vi "ABB Test Locked Rotor.vi"() -> ()   [LabVIEW 2017]
uses:
  Temp error msg.ctl
  Video Display Buttons.ctl
  ABB global.vi
panel:
  in  "Video Displays":T1
  in  "Temp error":T2="Error: Temperature measurement "
  out "Auto Readings":cluster{"%":dbl[], "Recorded":bool[]}
  in  "Simulate I":dbl(slide)
  out "Readings":string[][](table)
  out "In Range?":bool[](array[boolean])
  out "saved Readings":dbl[][](array[numeric])
  out "% rated current":dbl format="%.1f"
  out "Rated Current":dbl
  out "Serial number":string
  out "W.O number":string
  out "Power":string[][](table)
  out "Current & Voltage":string[][](table)
  out "Norma 5000 Error":string
  in  "Record":bool
  out "Readings":string[][](table)
  in  "View":enum16{"Graph", "Readings"}(ring)
  out "Number readings":i32
  out "Status":enum16{"Stopped", "Running"}(ring)
  out "Timedate":string
  in  "End test":bool
  in  "Start":bool
  in  "Read Mode":enum16{"Auto", "Manual"}(ring)
  in  "Exit":bool
  out "Current vs Voltage":T3(graph)
  # "Locked Rotor Test"
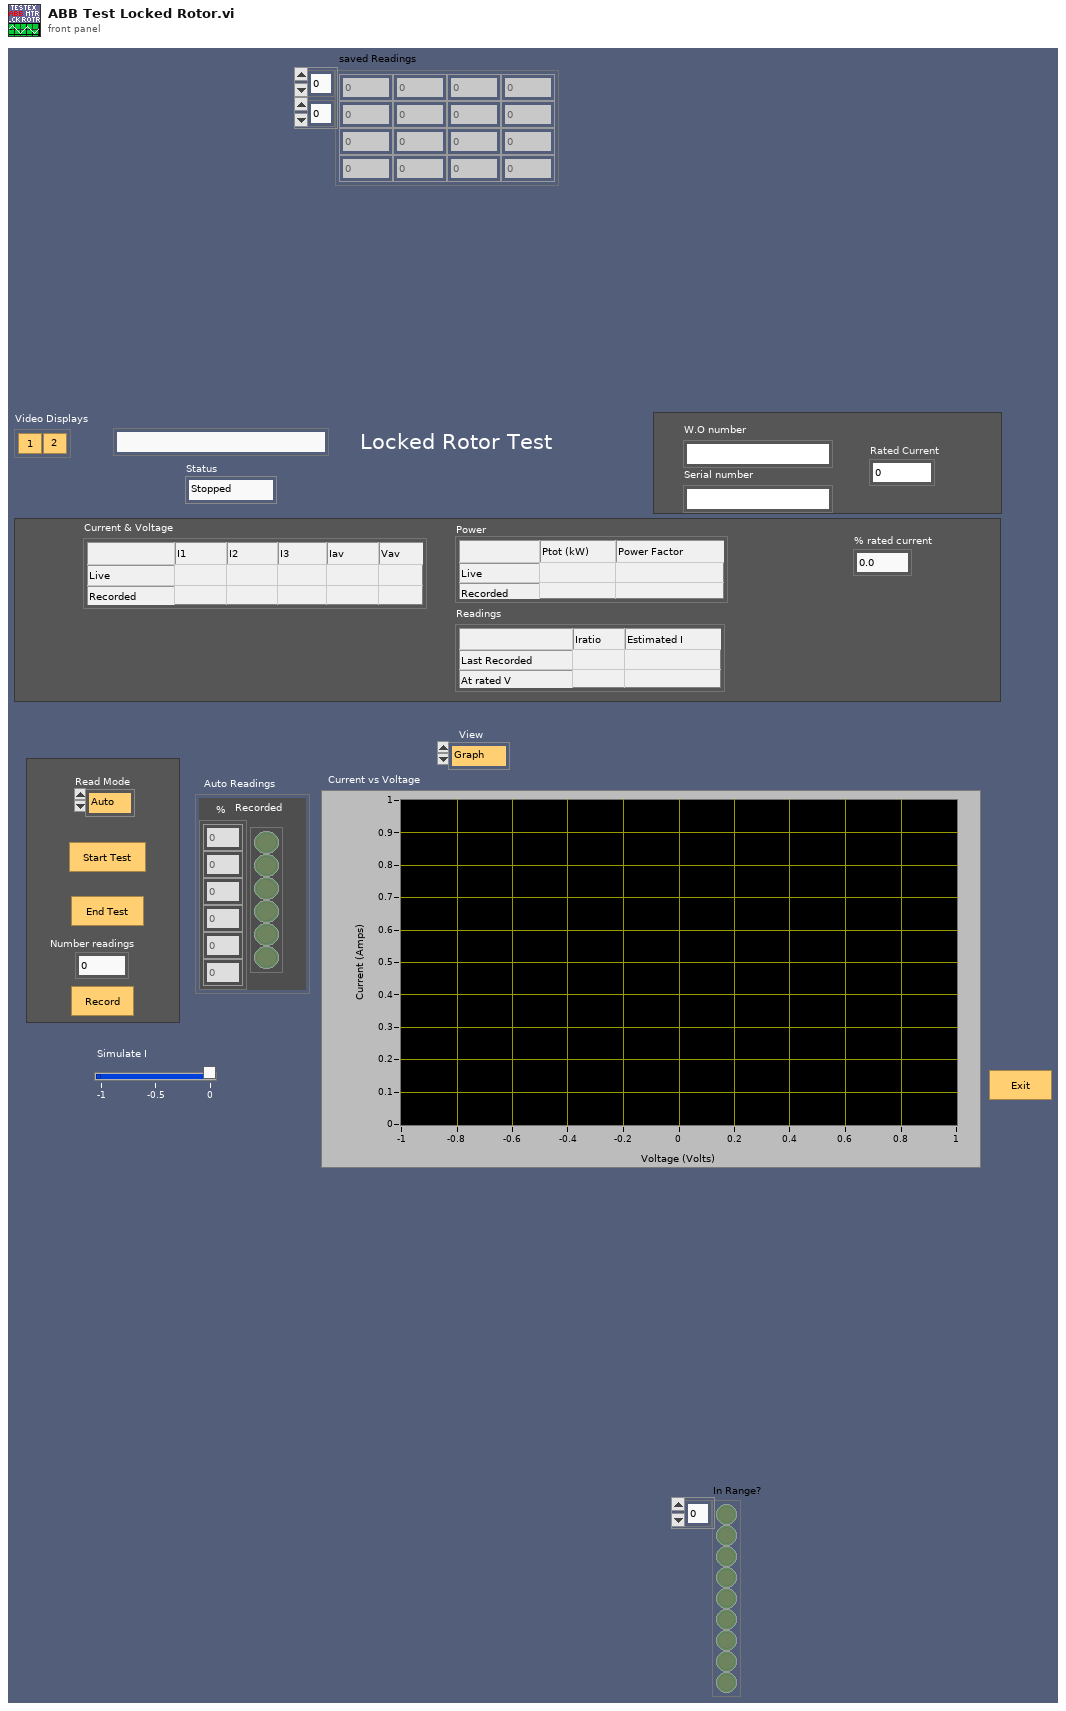
[diagram p1: front panel]
types:
  T1 = typedef "Video Display Buttons.ctl" = cluster{"1":bool, "1 2":bool}
  T2 = typedef "Temp error msg.ctl" = string
  T3 = cluster{"Sorted 2D Array":dbl[], "Sorted 2D Array":dbl[]}
  T4 = cluster{"Voltage":dbl, "Power":dbl, "Current":dbl, "PF":dbl}
  T5 = cluster{"VT Primary":dbl, "VT Secondary":dbl, "CT  Primary":dbl, "CT Secondary":dbl, "Current Shunt":enum16{"Internal", "External"}, "Avg interval":dbl}
  T6 = cluster{"VT Primary":dbl, "VT Secondary":dbl, "CT  Primary":dbl, "CT Secondary":dbl, "Current Shunt":enum16{"Internal", "External"}, "Averaging interval (secs)":dbl}
  T7 = cluster{"Visa sesssion":refnum<visa-resource-name>, "error":errorcluster}
  T8 = cluster{"Simulate Norma":bool, "Norma 5000 Address":u8, "WebDaq IP Address":string, "Simulate cDAQ":bool}
  T9 = cluster{"Number Values":i32, "Tolerance":dbl, "Value (ratio) ":dbl[], "Hold time (sec)":dbl}
  T10 = cluster{"V":dbl, "A":dbl, "W":dbl, "VA":dbl, "VAr":dbl, "Pf":dbl}
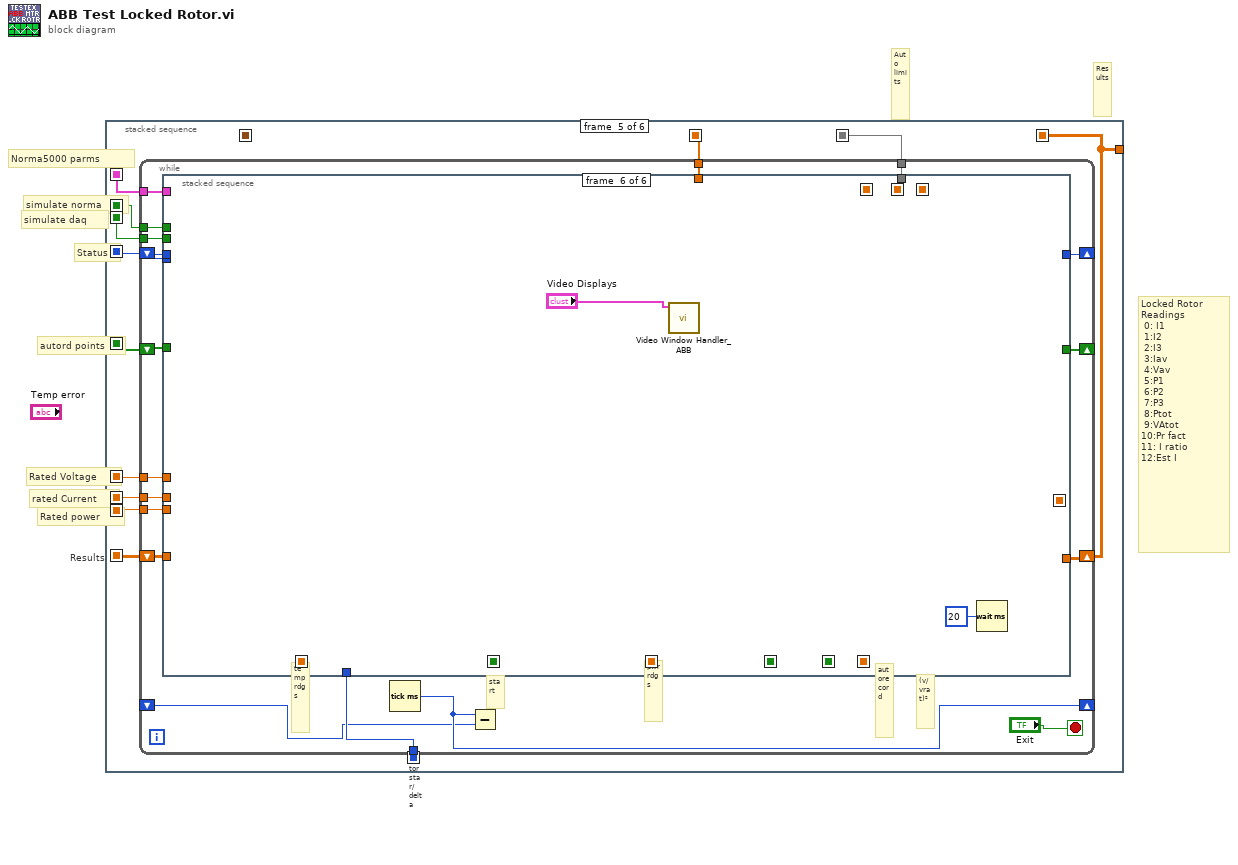
[diagram p0: block diagram]
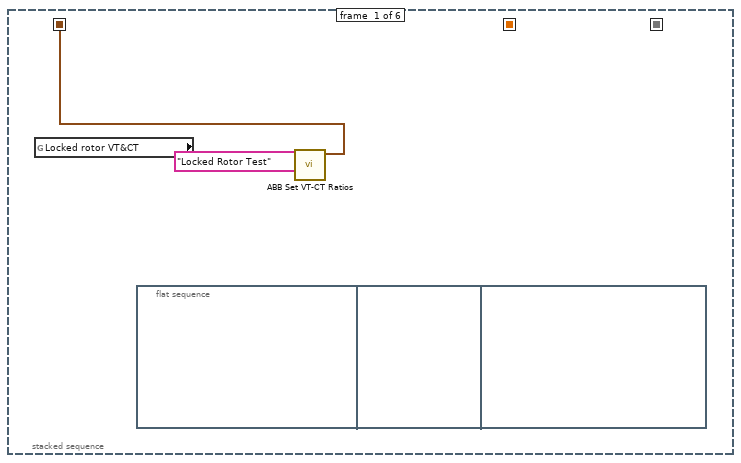
[diagram p2: hidden frame]
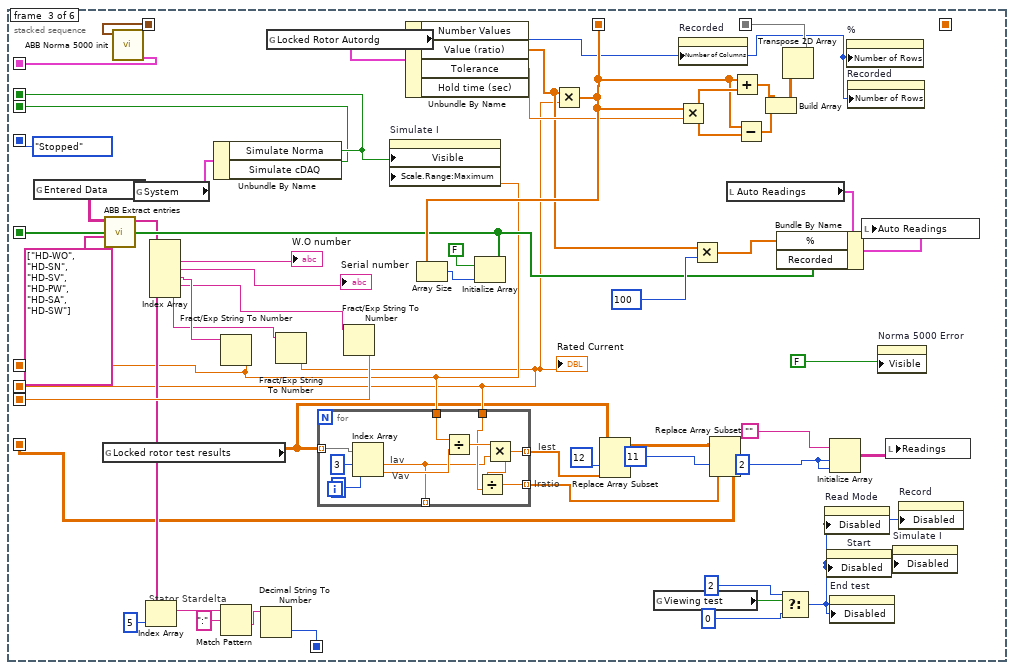
[diagram p4: hidden frame]
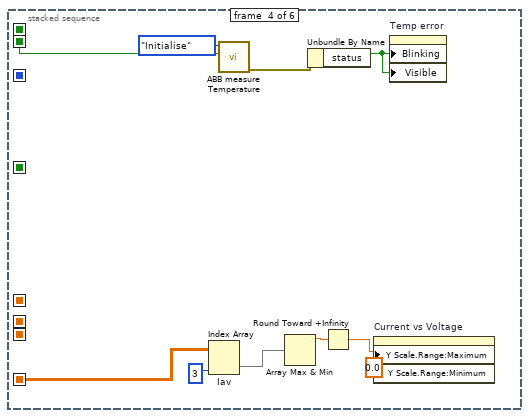
[diagram p5: hidden frame]
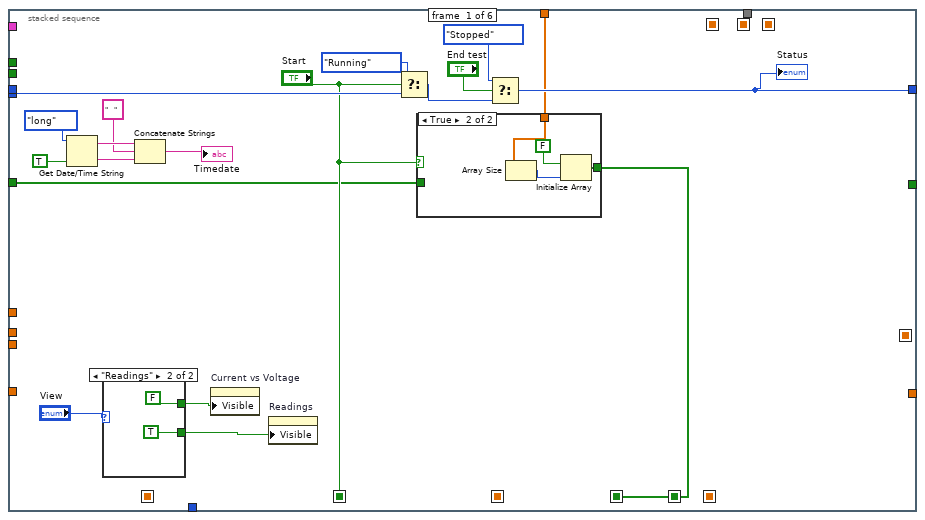
[diagram p6: hidden frame]
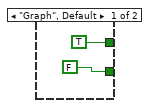
[diagram p8: hidden frame]
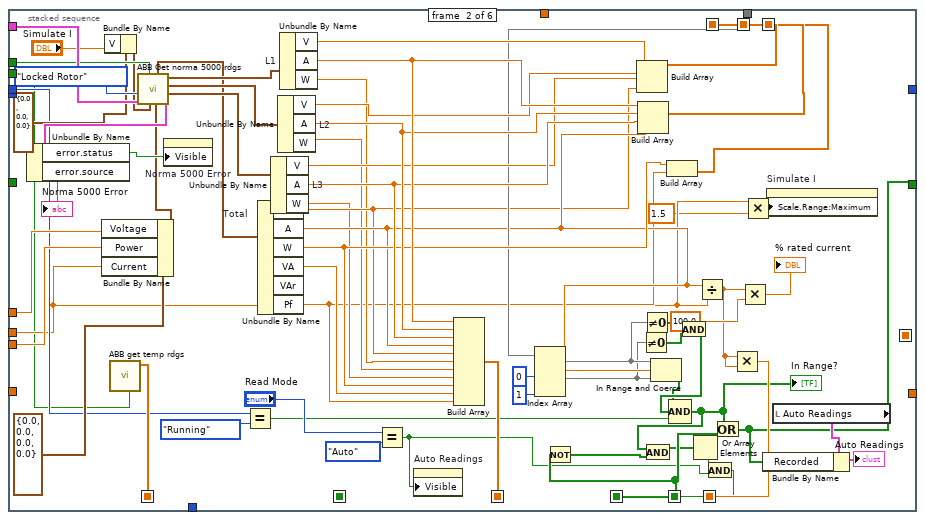
[diagram p9: hidden frame]
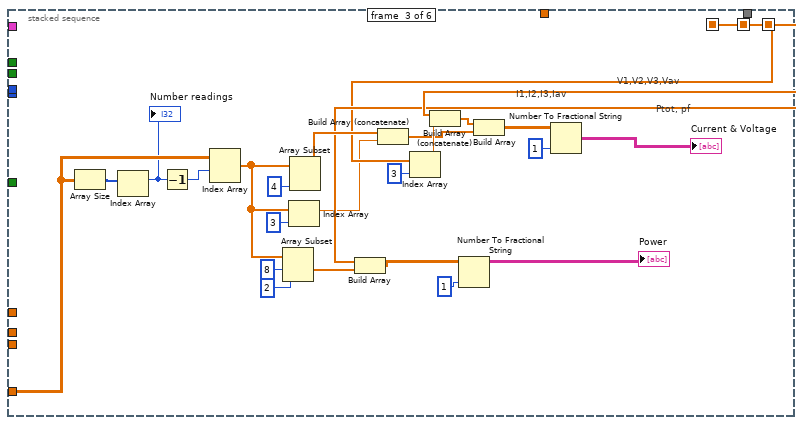
[diagram p10: hidden frame]
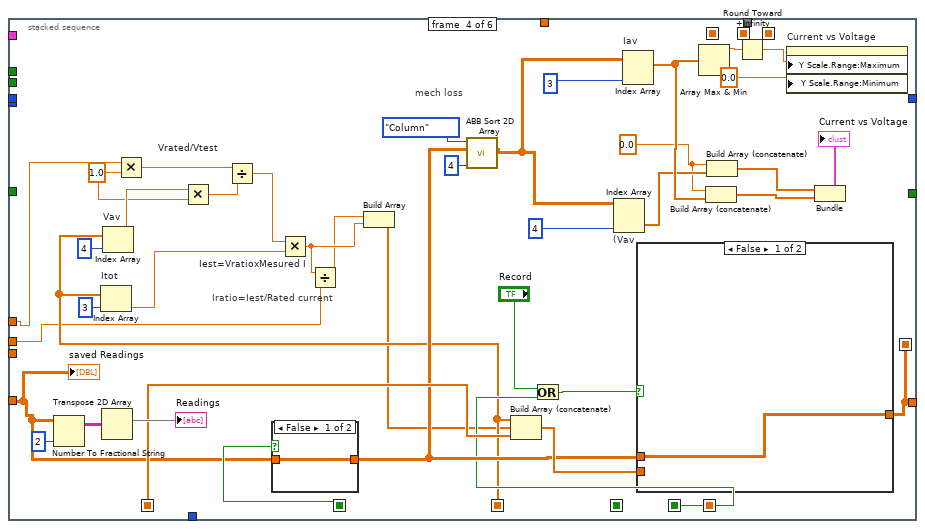
[diagram p11: hidden frame]
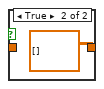
[diagram p12: hidden frame]
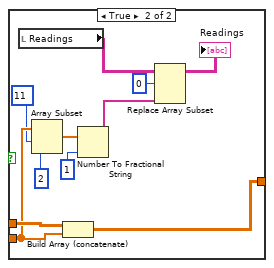
[diagram p13: hidden frame]
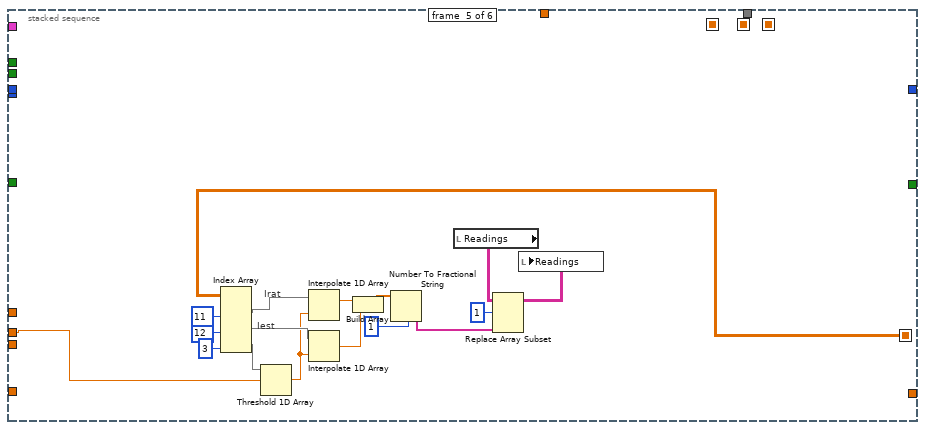
[diagram p14: hidden frame]
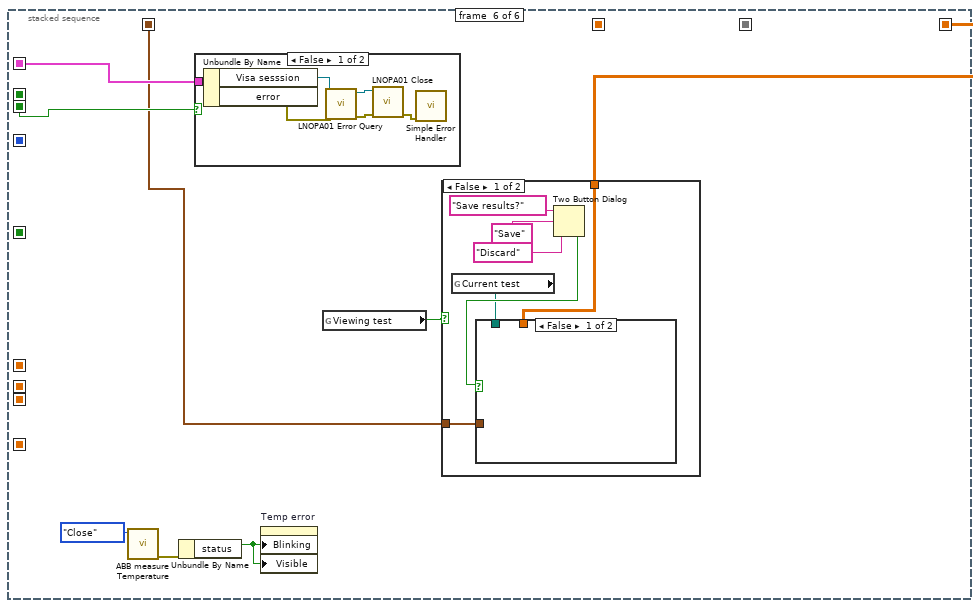
[diagram p15: hidden frame]
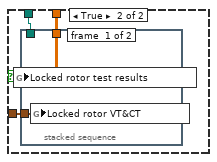
[diagram p16: hidden frame]
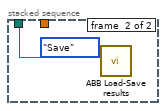
[diagram p17: hidden frame]
diagram:
  # "Results"
  # "stator star/delta"
  # "simulate daq"
  # "Results"
  # "Rated power"
  # "Rated Voltage"
  # "Locked Rotor\nReadings\n 0: I1\n 1:I2\n 2:I3\n 3:Iav\n 4:Vav\n 5:P1\n 6:P2\n 7:P3\n 8:Ptot\n 9:VAtot\n10:Pr fact\n11: I ratio\n12:Est I"
  # "autord points"
  # "Auto limits"
  # "rated Current"
  # "simulate norma"
  # "Norma5000 parms"
  # "Status"
  n1 = stacked-sequence {
    seq-local: [_ _ enum16{"Stopped", "Running"}."Stopped" ("Status") _ _ _] -> [_ _ _ _ w90 _]
    seq-local: [_ _ w56 _ _ _] -> [_ _ _ _ w89 w310]
    seq-local: [_ _ w42 _ _ _] -> [_ _ _ _ w88 w309]
    seq-local: [_ _ w11 _ _ _] -> [_ _ _ _ w87 _]
    seq-local: [_ _ w4 _ _ _] -> [_ _ _ w72 w86 _]
    seq-local: [_ _ w24 _ _ _] -> [_ _ _ _ w85 _]
    seq-local: [_ _ w48 _ _ _] -> [_ _ _ _ w83 _]
    seq-local: [_ _ w46 _ _ _] -> [_ _ _ _ w84 _]
    seq-local: [_ _ w12 _ _ _] -> [_ _ _ _ w82 _]
    seq-local: [_ _ w43 _ _ _] -> [_ _ _ _ w81 _]
    seq-local: [_ _ _ _ w78 _] -> [_ _ _ _ _ w307]
    seq-local: [_ _ w30 _ _ _] -> [_ _ _ w71 w79 _]
    seq-local: [_ _ w17 _ _ _] -> [_ _ _ _ w80 _]
    seq-local: [w1 _ _ _ _ _] -> [_ _ w13 _ _ w306]
    tunnel: [_ _ _ _ w78 _] -> _
    frame #0 {
      n2 = global read "ABB global.vi" "Locked rotor VT&CT"() -> (w3:T5)
      n3 = flat-sequence {
        frame #0 {
        }
        frame #1 {
        }
        frame #2 {
        }
      }
      n4 = call "ABB Set VT-CT Ratios.vi"("Test name"="Locked Rotor Test", "VT and CT Ratios"=w3) -> ("VT and CT Ratios out"=w1:T6)  [unwired: 9 in]
    }
    frame #1 {
    }
    frame #2 {
      w14 = 2
      # "Iratio"
      # "Iest"
      # "Stator Stardelta"
      n5 = global read "ABB global.vi" "Entered Data"() -> (w41:string[][])
      n6 = global read "ABB global.vi" "Locked rotor test results"() -> (w10:dbl[][])
      n7 = call "ABB Extract entries.vi"("Entry IDs"=string[] ["HD-WO", "HD-SN", "HD-SV", "HD-PW", "HD-SA", "HD-SW"], "Entry table in"=w41) -> ("Selected Entries"=w18:string[])  [unwired: 9 in]
      n8 = call "ABB Norma 5000 init.vi"("VT and CT Ratios"=w13) -> ("norma 5000 parms out"=w56:T7)  [unwired: 10 in]
      n9 = global read "ABB global.vi" "System"() -> (w55:T8)
      n10 = Index Array(array=w18, index=5) -> (element=w21:string)
      n11 = Index Array(array=w18) -> (element #1=→"W.O number":string, element #2=→"Serial number":string, element #3=w37:string, element #4=w36:string, element #5=w35:string)  [unwired: 5 in]
      n12 = Unbundle By Name(w55) -> ("Simulate Norma"=w42:bool, "Simulate cDAQ"=w30:bool)
      n13 = Fract/Exp String To Number(string=w37) -> (number=w12:dbl)  [unwired: 3 in, 1 out]
      n14 = Match Pattern(string=w21, regular expression=":") -> (after substring=w19:string)  [unwired: 1 in, 3 out]
      n15 = Decimal String To Number(string=w19) -> (number=w17:i32)  [unwired: 2 in, 1 out]
      n16 = global read "ABB global.vi" "Locked Rotor Autordg"() -> (w45:T9)
      n17 = Fract/Exp String To Number(string=w35) -> (number=w11:dbl)  [unwired: 3 in, 1 out]
      "Rated Current" <- w11
      n18 = for {
        tunnel: w10 -> [w67] mode=indexing
        tunnel: w12 -> [w63]
        tunnel: w11 -> [w61]
        tunnel: [w60] -> w8 mode=indexing
        tunnel: [w59] -> w7 mode=indexing
        tunnel: [w58] -> _ mode=indexing
        # "Vav"
        # "Iav"
        n19 = Index Array(array=w67, index #1=3 ("index"), index #2=4) -> (element #1=w58:dbl, element #2=w64:dbl)
        n20 = Divide(x=w63, y=w64) -> (x/y=w62:dbl)
        n21 = Multiply(x=w62, y=w58) -> (x*y=w60:dbl)
        n22 = Divide(x=w60, y=w61) -> (x/y=w59:dbl)
      }
      n23 = Fract/Exp String To Number(string=w36) -> (number=w43:dbl)  [unwired: 3 in, 1 out]
      n24 = property on="Simulate I" class="Slide (strict)"("Visible"=w42, "Scale.Range:Maximum"=w12) -> ()  [unwired: 2 in, 2 out]
      n25 = Unbundle By Name(w45) -> ("Number Values"=w23:i32, "Value (ratio)"=w29:dbl[], "Tolerance"=w44:dbl)  [unwired: 1 out]
      n26 = Multiply(x=w29, y=w11) -> (x*y=w46:dbl[])
      n27 = Array Size(array=w46) -> (size(s)=w53:i32)
      n28 = Initialize Array(FALSE, w53) -> (w24:bool[])
      n29 = Replace Array Subset(array=w10, new element=w8, index (col)=12 ("index (row)")) -> (w9:dbl[][])  [unwired: 1 in]
      n30 = global read "ABB global.vi" "Viewing test"() -> (w34:bool)
      n31 = Multiply(x=w46, y=w44) -> (x*y=w50:dbl[])
      n32 = property on="Recorded" class="Arr (strict)"("Number of Columns"=w23) -> ()  [unwired: 2 in, 2 out]
      n33 = Multiply(x=w29, y=100 ("Numeric")) -> (x*y=w25:dbl[])
      n34 = Replace Array Subset(array=w9, new element=w7, index (col)=11 ("index (row)")) -> (w4:dbl[][])  [unwired: 1 in]
      n35 = local read "Auto Readings"() -> (w27:cluster{"%":dbl[], "Recorded":bool[]})
      n36 = Add(x=w46, y=w50) -> (x+y=w51:dbl[])
      n37 = Subtract(x=w46, y=w50) -> (x-y=w47:dbl[])
      n38 = Build Array(w51, w47) -> (w49:dbl[][])
      n39 = Bundle By Name(cluster=w27, "%"=w25, "Recorded"=w24) -> (w26:cluster{"%":dbl[], "Recorded":bool[]})
      n40 = Select(t=2, s=w34, f=0) -> (s? t:f=w31:i32)
      n41 = Transpose 2D Array(2D array=w49) -> (transposed array=w48:dbl[][])
      n42 = property on="Read Mode" class="Enum (strict)"("Disabled"=w31) -> ()  [unwired: 2 in, 2 out]
      n43 = property on="Start" class="Bool"("Disabled"=w31) -> ()  [unwired: 2 in, 2 out]
      n44 = Initialize Array("", w14, w14) -> (w16:string[][])
      n45 = property on="End test" class="Bool"("Disabled"=w31) -> ()  [unwired: 2 in, 2 out]
      n46 = property on="%" class="Arr (strict)"("Number of Rows"=w23) -> ()  [unwired: 2 in, 2 out]
      n47 = property on="Recorded" class="Arr (strict)"("Number of Rows"=w23) -> ()  [unwired: 2 in, 2 out]
      n48 = local write "Auto Readings"(w26) -> ()
      n49 = property on="Norma 5000 Error" class="Str"("Visible"=FALSE) -> ()  [unwired: 2 in, 2 out]
      n50 = local write "Readings"(w16) -> ()
      n51 = property on="Simulate I" class="Slide (strict)"("Disabled"=w31) -> ()  [unwired: 2 in, 2 out]
      n52 = property on="Record" class="Bool"("Disabled"=w31) -> ()  [unwired: 2 in, 2 out]
    }
    frame #3 {
      n53 = Index Array "Iav"(array=w72, index (col)=3 ("disabled index (col)")) -> (element=w74:dbl[])  [unwired: 1 in]
      n54 = call "ABB measure Temperature.vi"("Simulate"=w71, "Mode"=enum16{"Initialise", "Read", "Close"}."Initialise") -> ("error out"=w69:errorcluster)  [unwired: 7 in, 2 out]
      n55 = Array Max & Min(array=w74) -> (max value=w77:dbl)  [unwired: 3 out]
      n56 = Unbundle By Name(w69) -> ("status"=w68:bool)
      n57 = Round Toward +Infinity(x=w77) -> (ceil(x): smallest int >= x=w73:dbl)
      n58 = property on="Current vs Voltage" class="XYGraph (strict)"("Y Scale.Range:Maximum"=w73, "Y Scale.Range:Minimum"=0.0) -> ()  [unwired: 2 in, 2 out]
      n59 = property on="Temp error" class="Str (strict)"("Blinking"=w68, "Visible"=w68) -> ()  [unwired: 2 in, 2 out]
    }
    frame #4 {
      n60 = while {
        shift-right: [w107] -> _
        shift-left: w90 -> [w95]
        tunnel: w89 -> [w106]
        tunnel: w88 -> [w105]
        tunnel: w87 -> [w104]
        shift-right: [w102] -> w78
        shift-left: w86 -> [w103]
        shift-right: [w101] -> _
        shift-left: w85 -> [w100]
        tunnel: w84 -> [w99]
        tunnel: w83 -> [w98]
        tunnel: w82 -> [w97]
        tunnel: w81 -> [w96]
        tunnel: w80 -> [w94]
        tunnel: w79 -> [w93]
        shift-right: [w92] -> _
        shift-left: _ -> [w91]
        stop <- "Exit" stop-if-true
        # "autorecord"
        # "(v/vrat)²"
        # "temp rdgs"
        # "pwr rdgs"
        # "start"
        n61 = stacked-sequence {
          seq-local: ["Start" _ _ _ _ _] -> [_ _ _ w269 _ _]
          seq-local: [_ w186 _ _ _ _] -> [_ _ _ w252 _ _]
          seq-local: [_ w185 _ _ _ _] -> [_ _ _ w263 _ _]
          seq-local: [_ w183 _ _ _ _] -> [_ _ _ _ _ _]
          seq-local: [w109 _ _ _ _ _] -> [_ w179 _ _ _ _]
          seq-local: [_ w177 _ _ _ _] -> [_ _ _ w255 _ _]
          seq-local: [_ w174 _ _ _ _] -> [_ _ w209 _ _ _]
          seq-local: [_ w173 _ _ _ _] -> [_ _ w223 _ _ _]
          seq-local: [_ w172 _ _ _ _] -> [_ _ w215 _ _ _]
          seq-local: [_ _ _ w233 _ _] -> [_ _ _ _ w300 _]
          tunnel: w95 -> [w121 _ _ _ _ _]
          tunnel: [w116 _ _ _ _ _] -> w107
          tunnel: w106 -> [_ w204 _ _ _ _]
          tunnel: w105 -> [_ w196 _ _ _ _]
          tunnel: w104 -> [_ w153 _ w231 w295 _]
          tunnel: w103 -> [_ _ w228 w235 _ _]
          tunnel: [_ _ _ w233 _ _] -> w102
          tunnel: [_ w147 _ _ _ _] -> w101
          tunnel: w100 -> [w111 _ _ _ _ _]
          tunnel: w99 -> [w110 _ _ _ _ _]
          tunnel: w98 -> [_ w182 _ _ _ _]
          tunnel: w97 -> [_ w163 _ w241 _ _]
          tunnel: w96 -> [_ w162 _ _ _ _]
          tunnel: w95 -> [_ w156 _ _ _ _]
          tunnel: w94 -> [_ _ _ _ _ _]
          tunnel: w93 -> [_ w137 _ _ _ _]
          frame #0 {
            n62 = Get Date/Time String(date format (0)=enum16{"short", "long", "abbreviated"}."long", want seconds? (F)=TRUE) -> (date string=w125:string, time string=w124:string)  [unwired: 1 in]
            n63 = case shown="\"Readings\"" "View" {
              tunnel: [TRUE FALSE] -> w114
              tunnel: [FALSE TRUE] -> w113
              frame "Graph", Default {
              }
              frame "Readings" {
              }
            }
            n64 = Concatenate Strings(w125, "   ", w124) -> (→"Timedate":string)
            n65 = property on="Current vs Voltage" class="XYGraph (strict)"("Visible"=w114) -> ()  [unwired: 2 in, 2 out]
            n66 = property on="Readings" class="Tbl (strict)"("Visible"=w113) -> ()  [unwired: 2 in, 2 out]
            n67 = Select(t=enum16{"Stopped", "Running"}."Running", s="Start", f=w121) -> (s? t:f=w119:enum16{"Stopped", "Running"})
            n68 = case shown="True" "Start" {
              tunnel: w110 -> [_ w132]
              tunnel: [w128 w129] -> w109
              tunnel: w111 -> [w128 _]
              frame False {
              }
              frame True {
                n69 = Array Size(array=w132) -> (size(s)=w131:i32)
                n70 = Initialize Array(FALSE, w131) -> (w129:bool[])
              }
            }
            n71 = Select(t=enum16{"Stopped", "Running"}."Stopped", s="End test", f=w119) -> (s? t:f=w116:enum16{"Stopped", "Running"})
            "Status" <- w116
          }
          frame #1 {
            n72 = Bundle By Name(cluster=T4 {"Voltage"=0.0, "Power"=0.0, "Current"=0.0, "PF"=0.0} ("Rated"), "Voltage"=w163, "Power"=w162, "Current"=w153) -> (w161:T4)
            n73 = Bundle By Name(cluster=cluster{"V":dbl, "A":dbl, "pwr factor":dbl} {"V"=0.0, "A"=0.0, "pwr factor"=0.0} ("Simulation rdgs"), "V"="Simulate I") -> (w158:cluster{"V":dbl, "A":dbl, "pwr factor":dbl})
            n74 = call "ABB get temp rdgs.vi"("Sim daq"=w137) -> ("Category rdgs"=w185:dbl[])  [unwired: 7 in, 3 out]
            n75 = call "ABB Get norma 5000 rdgs.vi"("Rated"=w161, "Simulation rdgs"=w158, "simulate"=w196, "norma 5000 parms in"=w204, "Simulate Mode"=enum16{"No load", "Locked Rotor"}."Locked Rotor") -> ("norma 5000 parms out"=w198:T7, "L 3"=w199:T10, "L 2"=w200:T10, "L1"=w201:T10, "Total"=w197:T10)  [unwired: 2 in]
            n76 = Unbundle By Name(w198) -> ("error.status"=w203:bool, "error.source"=→"Norma 5000 Error":string)
            n77 = property on="Norma 5000 Error" class="Str"("Visible"=w203) -> ()  [unwired: 2 in, 2 out]
            n78 = Equal?(x=w156, y=enum16{"Stopped", "Running"}."Running") -> (x = y?=w154:bool)
            n79 = Unbundle By Name "Total"(w197) -> ("V"=w170:dbl, "A"=w171:dbl, "W"=w187:dbl, "VA"=w166:dbl, "Pf"=w165:dbl)  [unwired: 1 out]
            n80 = Unbundle By Name "L3"(w199) -> ("V"=w188:dbl, "A"=w191:dbl, "W"=w167:dbl)
            n81 = Unbundle By Name "L2"(w200) -> ("V"=w189:dbl, "A"=w192:dbl, "W"=w168:dbl)
            n82 = Unbundle By Name "L1"(w201) -> ("V"=w190:dbl, "A"=w193:dbl, "W"=w169:dbl)
            n83 = Equal?(x="Read Mode", y=enum16{"Auto", "Manual"}."Auto") -> (x = y?=w150:bool)
            n84 = property on="Auto Readings" class="Clust (strict)"("Visible"=w150) -> ()  [unwired: 2 in, 2 out]
            n85 = Build Array(w193, w192, w191, w171, w170, w169, w168, w167, w187, w166, w165) -> (w186:dbl[])
            n86 = Index Array(array=w182, index (col) #1=0 ("disabled index (col)"), index (col) #2=1 ("index (col)")) -> (element #1=w144:dbl[], element #2=w143:dbl[])  [unwired: 2 in]
            n87 = Not(x=w179) -> (.not. x?=w141:bool[])
            n88 = Build Array(w190, w189, w188, w170) -> (w174:dbl[])
            n89 = Build Array(w193, w192, w191, w171) -> (w173:dbl[])
            n90 = Not Equal To 0?(x=w143) -> (x != 0?=w145:bool[])
            n91 = Not Equal To 0?(x=w144) -> (x != 0?=w146:bool[])
            n92 = In Range and Coerce(upper limit=w144, x=w171, lower limit=w143) -> (In Range?=w140:bool[])  [unwired: 1 out]
            n93 = Build Array(w187, w165) -> (w172:dbl[])
            n94 = And(x=w146, y=w145) -> (x .and. y?=w142:bool[])
            n95 = Compound Arithmetic op=AND(w140, w142, w154) -> (w138:bool[])
            "In Range?" <- w138
            n96 = And(x=w138, y=w141) -> (x .and. y?=w139:bool[])
            n97 = Or Array Elements(Boolean array=w139) -> (logical OR=w178:bool)
            n98 = Divide(x=w171, y=w153) -> (x/y=w184:dbl)
            n99 = And(x=w178, y=w150) -> (x .and. y?=w177:bool)
            n100 = Or(x=w138, y=w179) -> (x .or. y?=w147:bool[])
            n101 = Multiply(x=w184, y=w184) -> (x*y=w183:dbl)
            n102 = Multiply(x=w184, y=100.0) -> (x*y=→"% rated current":dbl)
            n103 = Multiply(x=w153, y=1.5) -> (x*y=w151:dbl)
            n104 = property on="Simulate I" class="Slide (strict)"("Scale.Range:Maximum"=w151) -> ()  [unwired: 2 in, 2 out]
            n105 = local read "Auto Readings"() -> (w149:cluster{"%":dbl[], "Recorded":bool[]})
            n106 = Bundle By Name(cluster=w149, "Recorded"=w147) -> (→"Auto Readings":cluster{"%":dbl[], "Recorded":bool[]})
          }
          frame #2 {
            # "I1,I2,I3,Iav"
            # "V1,V2,V3,Vav"
            # "Ptot, pf"
            n107 = Array Size(array=w228) -> (size(s)=w229:i32[])
            n108 = Index Array(array=w229) -> (element=w212:i32)  [unwired: 1 in]
            "Number readings" <- w212
            n109 = Decrement(x=w212) -> (x-1=w227:i32)
            n110 = Index Array(array=w228, index (row)=w227) -> (element=w213:dbl[])  [unwired: 1 in]
            n111 = Array Subset(array=w213, index=8, length=2) -> (w216:dbl[])
            n112 = Index Array(array=w213, index=3) -> (element=w205:dbl)
            n113 = Array Subset(array=w213, length=4) -> (w222:dbl[])  [unwired: 1 in]
            n114 = Build Array(w215, w216) -> (w217:dbl[][])
            n115 = Build Array (concatenate)(w222, w205) -> (w207:dbl[])
            n116 = Index Array(array=w209, index=3) -> (element=w208:dbl)
            n117 = Build Array (concatenate)(w223, w208) -> (w210:dbl[])
            n118 = Number To Fractional String(number=w217, precision (6)=i16 1) -> (F-format string=→"Power":string[][])  [unwired: 2 in]
            n119 = Build Array(w210, w207) -> (w221:dbl[][])
            n120 = Number To Fractional String(number=w221, precision (6)=i16 1) -> (F-format string=→"Current & Voltage":string[][])  [unwired: 2 in]
          }
          frame #3 {
            w234 = 1.0 ("y")
            w236 = 0.0
            # "Iratio=Iest/Rated current"
            # "mech loss"
            n121 = Number To Fractional String(number=w235, precision (6)=i16 2) -> (F-format string=w268:string[][])  [unwired: 2 in]
            n122 = Index Array "Itot"(array=w252, index=3) -> (element=w240:dbl)
            n123 = Transpose 2D Array(2D array=w268) -> (transposed array=→"Readings":string[][])
            n124 = Index Array "Vav"(array=w252, index=4) -> (element=w244:dbl)
            n125 = Multiply(x=w241, y=w234) -> (x*y=w242:dbl)
            n126 = Multiply(x=w244, y=w234) -> (x*y=w243:dbl)
            n127 = Divide "Vrated/Vtest"(x=w242, y=w243) -> (x/y=w246:dbl)
            n128 = case shown="False" w269 {
              tunnel: w235 -> [w270 _]
              tunnel: [w270 dbl[][] []] -> w257
              frame False {
              }
              frame True {
              }
            }
            n129 = Multiply "Iest=VratioxMesured I"(x=w246, y=w240) -> (x*y=w232:dbl)
            n130 = Divide(x=w232, y=w231) -> (x/y=w230:dbl)
            n131 = Build Array(w230, w232) -> (w245:dbl[])
            n132 = call "ABB Sort 2D Array.vi"("Column/Row to Sort By"=u32 4, "Unsorted 2D Array"=w257, "Sort by"=enum16{"Column", "Row"}."Column") -> ("Sorted 2D Array"=w250:dbl[][])  [unwired: 4 in]
            n133 = Build Array (concatenate)(w252, w245, w263) -> (w264:dbl[])
            n134 = Or(x="Record", y=w255) -> (x .or. y?=w256:bool)
            n135 = Index Array "(Vav"(array=w250, index (col)=4 ("disabled index (col)")) -> (element=w247:dbl[])  [unwired: 1 in]
            n136 = Index Array "Iav"(array=w250, index (col)=3 ("disabled index (col)")) -> (element=w249:dbl[])  [unwired: 1 in]
            n137 = case shown="False" w256 {
              tunnel: w257 -> [w272 w283]
              tunnel: [w272 w282] -> w233
              tunnel: w264 -> [_ w277]
              frame False {
              }
              frame True {
                n138 = local read "Readings"() -> (w280:string[][])
                n139 = Array Subset(array=w277, index=11, length=2) -> (w274:dbl[])
                n140 = Build Array (concatenate)(w283, w277) -> (w282:dbl[][])
                n141 = Number To Fractional String(number=w274, precision (6)=i16 1) -> (F-format string=w273:string[])  [unwired: 2 in]
                n142 = Replace Array Subset(array=w280, new element=w273, index (row)=0) -> (→"Readings":string[][])  [unwired: 1 in]
              }
            }
            n143 = Array Max & Min(array=w249) -> (max value=w260:dbl)  [unwired: 3 out]
            n144 = Build Array (concatenate)(w236, w249) -> (w237:dbl[])
            n145 = Build Array (concatenate)(w236, w247) -> (w238:dbl[])
            n146 = Round Toward +Infinity(x=w260) -> (ceil(x): smallest int >= x=w248:dbl)
            n147 = property on="Current vs Voltage" class="XYGraph (strict)"("Y Scale.Range:Maximum"=w248, "Y Scale.Range:Minimum"=0.0) -> ()  [unwired: 2 in, 2 out]
            n148 = Bundle(w238, w237) -> (→"Current vs Voltage":cluster{dbl[], dbl[]})  [unwired: 1 in]
            "saved Readings" <- w235
          }
          frame #4 {
            # "Iest"
            # "Irat"
            n149 = Index Array(array=w300, index (col) #1=11 ("disabled index (col)"), index (col) #2=12 ("index (col)"), index (col) #3=3 ("index (col)")) -> (element #1=w294:dbl[], element #2=w293:dbl[], element #3=w296:dbl[])  [unwired: 3 in]
            n150 = Threshold 1D Array(2:w295, 3:w296) -> (0:w292:dbl)  [unwired: 1 in]
            n151 = Interpolate 1D Array(1:w292, 2:w294) -> (0:w287:dbl)
            n152 = Interpolate 1D Array(1:w292, 2:w293) -> (0:w286:dbl)
            n153 = Build Array(w287, w286) -> (w285:dbl[])
            n154 = Number To Fractional String(number=w285, precision (6)=i16 1) -> (F-format string=w284:string[])  [unwired: 2 in]
            n155 = local read "Readings"() -> (w290:string[][])
            n156 = Replace Array Subset(array=w290, new element=w284, index (row)=1) -> (w289:string[][])  [unwired: 1 in]
            n157 = local write "Readings"(w289) -> ()
          }
          frame #5 {
            n158 = call "Video Window Handler_ABB.vi"("Video Displays"="Video Displays") -> ()  [unwired: 11 in]
            n159 = Wait (ms)(milliseconds to wait=u32 20) -> ()  [unwired: 1 out]
          }
        }
        n160 = Tick Count (ms)() -> (millisecond timer value=w92:u32)
        n161 = Subtract(x=w92, y=w91) -> ()  [unwired: 1 out]
      }
    }
    frame #5 {
      n162 = call "ABB measure Temperature.vi"("Mode"=enum16{"Initialise", "Read", "Close"}."Close") -> ("error out"=w303:errorcluster)  [unwired: 8 in, 2 out]
      n163 = Unbundle By Name(w303) -> ("status"=w304:bool)
      n164 = case shown="False" w309 {
        tunnel: w310 -> [w327 _]
        frame False {
          n165 = Unbundle By Name(w327) -> ("Visa sesssion"=w326:refnum<visa-resource-name>, "error"=w325:errorcluster)
          n166 = call "LNOPA01 Error Query.vi"("error in (no error)"=w325, "VISA session"=w326) -> ("error out"=w328:errorcluster, "dup VISA session"=w329:refnum<visa-resource-name>)  [unwired: 6 in, 2 out]
          n167 = call "LNOPA01 Close.vi"("error in (no error)"=w328, "VISA session"=w329) -> ("error out"=w330:errorcluster)  [unwired: 9 in]
          n168 = call <vilib>:"Simple Error Handler.vi"("error in (no error)"=w330) -> ()  [unwired: 4 in, 5 out]
        }
        frame True {
        }
      }
      n169 = property on="Temp error" class="Str (strict)"("Blinking"=w304, "Visible"=w304) -> ()  [unwired: 2 in, 2 out]
      n170 = global read "ABB global.vi" "Viewing test"() -> (w308:bool)
      n171 = case shown="False" w308 {
        tunnel: w307 -> [w315 _]
        tunnel: w306 -> [w311 _]
        frame False {
          n172 = global read "ABB global.vi" "Current test"() -> (w314:path)
          n173 = Two Button Dialog(message="Save results?", 1:"Discard" ("F button name (\"Cancel\")"), 2:"Save" ("T button name (\"OK\")")) -> (T button?=w316:bool)
          n174 = case shown="False" w316 {
            tunnel: w315 -> [_ w320]
            tunnel: w314 -> [_ w319]
            tunnel: w311 -> [_ w318]
            frame False {
            }
            frame True {
              n175 = stacked-sequence {
                tunnel: w320 -> [w322 _]
                tunnel: w319 -> [_ w323]
                tunnel: w318 -> [w321 _]
                frame #0 {
                  n176 = global write "ABB global.vi" "Locked rotor test results"(w322) -> ()
                  n177 = global write "ABB global.vi" "Locked rotor VT&CT"(w321) -> ()
                }
                frame #1 {
                  n178 = call "ABB Load-Save results.vi"("Path"=w323, "Mode"=enum16{"LOAD", "Save"}."Save") -> ()  [unwired: 10 in]
                }
              }
            }
          }
        }
        frame True {
        }
      }
    }
  }
